vi "SQL Query.vi"(8 "error in (no error)":errorcluster, 10 "SQL Query":string, 11 "Database File":string) -> (0 "error out":errorcluster, 2 "Query Result":string, 3 "return code":i16)   [LabVIEW 2011]
doc: "Provides a simple query API to SQLite. The return code is determined by the SQLite Engine, and could be used to genertate a custom LabVIEW error. For more information on the SQLite query formats and erorrs please search to the SQLite documentation."
uses:
  SQLite Source/CVI RT/sqlitewrapper.dll
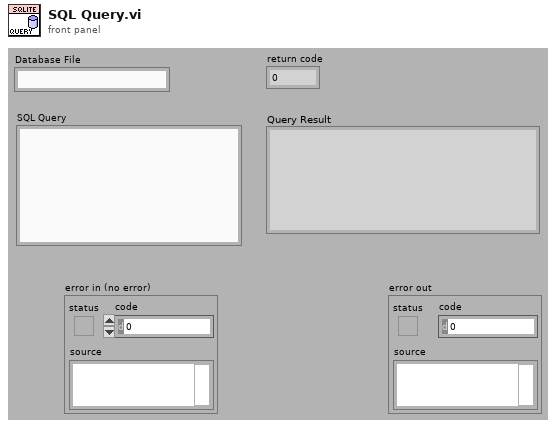
[diagram p1: front panel]
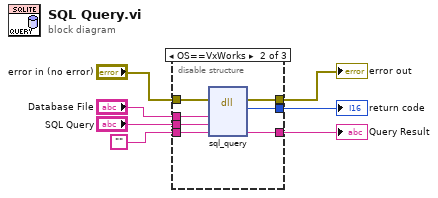
[diagram p0: block diagram]
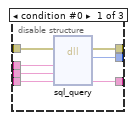
[diagram p2: hidden frame]
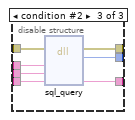
[diagram p3: hidden frame]
diagram:
  n1 = disable-structure shown="OS==VxWorks" {
    disable-tunnel: "Database File" -> [w14 w19 w26]
    disable-tunnel: "SQL Query" -> [w13 w18 w25]
    disable-tunnel: [w12 w15 w23] -> w5
    disable-tunnel: [w11 w16 w22] -> w4
    disable-tunnel: "" -> [w10 w17 w24]
    disable-tunnel: "error in (no error)" -> [w9 w20 w28]
    disable-tunnel: [w8 w21 w27] -> w1
    frame condition #0 {
      n2 = dll-call lib="C:/Git/B2G/lv_sqlite_103/SQLite Source/CVI RT/sqlitewrapper.*" fn="sql_query"(error in=w9, "dbfile"=w14, "query"=w13, "result"=w10) -> (error out=w8:errorcluster, "return type"=w11:i16, "result"=w12:string)  [unwired: 4 in, 1 out]
    }
    frame condition #1 (active) {
      n3 = dll-call lib="C:/Git/B2G/lv_sqlite_103/SQLite Source/CVI RT/sqlitewrapper.*" fn="sql_query"(error in=w20, "dbfile"=w19, "query"=w18, "result"=w17) -> (error out=w21:errorcluster, "return type"=w16:i16, "result"=w15:string)  [unwired: 4 in, 1 out]
    }
    frame condition #2 {
      n4 = dll-call lib="C:/Git/B2G/lv_sqlite_103/SQLite Source/CVI RT/sqlitewrapper.dll" fn="sql_query"(error in=w28, "dbfile"=w26, "query"=w25, "result"=w24) -> (error out=w27:errorcluster, "return type"=w22:i16, "result"=w23:string)  [unwired: 4 in, 1 out]
    }
  }
  "Query Result" <- w5
  "return code" <- w4
  "error out" <- w1
